vi "broadcastHPFreezeSensorValues.vi"(8 "error in (no error)":errorcluster, 9 "TriggerIRQ":bool, 10 "WaitForTrigger":bool, 11 "ILCCommunications in":refnum<class "ILCCommunications.lvclass">) -> (0 "error out":errorcluster, 3 "ILCCommunications out":refnum<class "ILCCommunications.lvclass">)   [LabVIEW 2016, in "ILCCommunications.lvclass"]
uses:
  ILCCommunications.lvclass
  ILCCommunications.lvclass/ILCCommunications.ctl
  Common_RT_Modbus/IModbus/IModbus.lvclass
  Common_RT_HPILC/HPILC/HPILC.lvclass
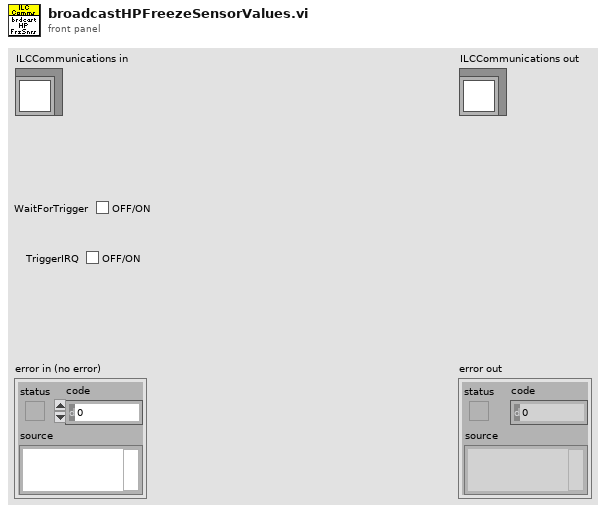
[diagram p1: front panel]
types:
  T1 = typedef "RTModbus.lvlib/TxFrame.ctl" = cluster{"Data":u8[], "WaitForTrigger":bool, "WaitForRx":u16, "TriggerIRQ":bool, "DelayMicroseconds":u16, "DelayMilliseconds":u16, "Timestamp":bool}
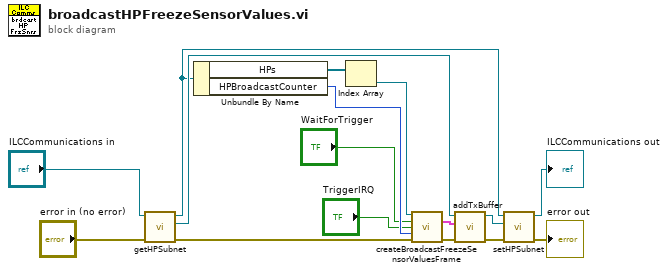
[diagram p0: block diagram]
diagram:
  n1 = call "getHPSubnet.vi"("error in (no error)"="error in (no error)", "ILCCommunications in"="ILCCommunications in") -> ("error out"=w11:errorcluster, "Modbus"=w10:refnum<class "IModbus.lvclass">, "ILCCommunications out"=w5:refnum<class "ILCCommunications.lvclass">)  [unwired: 7 in]
  n2 = Unbundle By Name(w5) -> ("HPs"=w13:refnum<class "HPILC.lvclass">[], "HPBroadcastCounter"=w15:u8)
  n3 = Index Array(array=w13) -> (element=w14:refnum<class "HPILC.lvclass">)  [unwired: 1 in]
  n4 = call "createBroadcastFreezeSensorValuesFrame.vi"("HPILC in"=w14, "WaitForTrigger"="WaitForTrigger", "TriggerIRQ"="TriggerIRQ", "BroadcastCounter"=w15, "error in (no error)"=w11) -> ("TxFrame"=w2:T1, "error out"=w1:errorcluster)  [unwired: 8 in, 1 out]
  n5 = call-dynamic "addTxBuffer.vi"("error in (no error)"=w1, "TxFrame"=w2, "IModbus in"=w10) -> ("error out"=w7:errorcluster, "IModbus out"=w9:refnum<class "IModbus.lvclass">)  [unwired: 7 in]
  n6 = call "setHPSubnet.vi"("error in (no error)"=w7, "Modbus"=w9, "ILCCommunications in"=w5) -> ("error out"=→"error out":errorcluster, "ILCCommunications out"=→"ILCCommunications out":refnum<class "ILCCommunications.lvclass">)  [unwired: 7 in]
